vi "LogRelayData.vi"(0 "Path":path, 2 "XCorr":i32, 3 "YCorr":i32, 5 "Rotation":dbl, 7 "Texp":dbl, 9 "CenX":dbl format="%.2f", 11 "CenY":dbl format="%.2g", 13 "XHex":dbl format="%.4f", 14 "YHex":dbl format="%.4f") -> ()   [LabVIEW 2011]
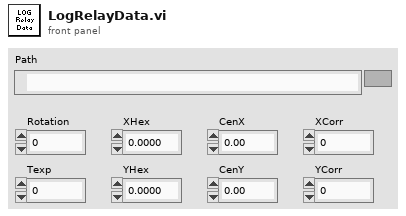
[diagram p1: front panel]
types:
  T1 = enum16{"open", "replace", "create", "open or create", "replace or create", "replace or create with confirmation"}
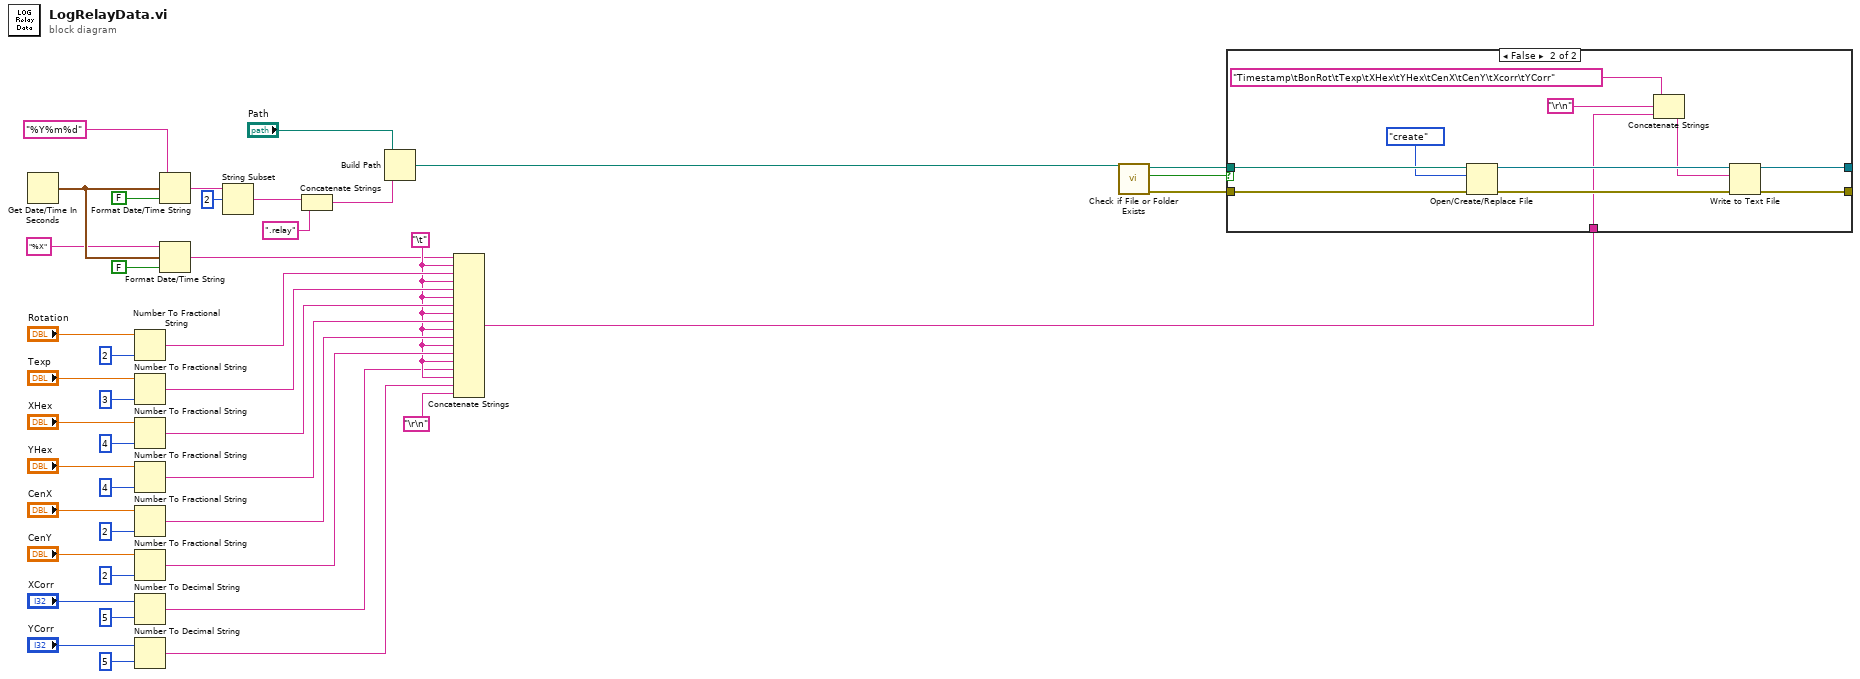
[diagram p0: block diagram]
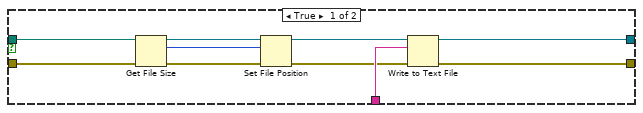
[diagram p2: hidden frame]
diagram:
  w12 = "\t"
  n1 = Get Date/Time In Seconds() -> (seconds since 1Jan1904=w42:timestamp)
  n2 = Number To Fractional String(number="Rotation", precision (6)=i16 2) -> (F-format string=w30:string)  [unwired: 2 in]
  n3 = Number To Fractional String(number="Texp", precision (6)=i16 3) -> (F-format string=w27:string)  [unwired: 2 in]
  n4 = Number To Fractional String(number="XHex", precision (6)=i16 4) -> (F-format string=w16:string)  [unwired: 2 in]
  n5 = Number To Fractional String(number="YHex", precision (6)=i16 4) -> (F-format string=w15:string)  [unwired: 2 in]
  n6 = Number To Fractional String(number="CenX", precision (6)=i16 2) -> (F-format string=w14:string)  [unwired: 2 in]
  n7 = Number To Fractional String(number="CenY", precision (6)=i16 2) -> (F-format string=w13:string)  [unwired: 2 in]
  n8 = Number To Decimal String(number="XCorr", width (-)=i16 5) -> (decimal integer string=w11:string)
  n9 = Number To Decimal String(number="YCorr", width (-)=i16 5) -> (decimal integer string=w10:string)
  n10 = Format Date/Time String(time format string (%c)="%Y%m%d", seconds (now)=w42, UTC format=FALSE) -> (date/time string=w38:string)
  n11 = Format Date/Time String(time format string (%c)="%X", seconds (now)=w42, UTC format=FALSE) -> (date/time string=w2:string)
  n12 = String Subset(string=w38, offset (0)=2) -> (substring=w35:string)  [unwired: 1 in]
  n13 = Concatenate Strings(w35, ".relay" ("string")) -> (w33:string)
  n14 = Build Path(base path="Path", name or relative path=w33) -> (appended path=w5:path)
  n15 = Concatenate Strings(w2, w12, w30, w12, w27, w12, w16, w12, w15, w12, w14, w12, w13, w12, w11, w12, w10, "\r\n") -> (w1:string)
  n16 = call <vilib>:"Check if File or Folder Exists.vi"("path"=w5) -> ("error out"=w8:errorcluster, "file or folder exists?"=w6:bool, "dup path"=w7:path)  [unwired: 8 in]
  n17 = case shown="False" w6 {
    tunnel: w7 -> [w47 w64]
    tunnel: w8 -> [w46 w63]
    tunnel: [w53 w62] -> _
    tunnel: [w52 w61] -> _
    tunnel: w1 -> [w51 w55]
    frame True {
      n18 = Get File Size(file=w47, error in=w46) -> (refnum out=w50:refnum<file>, size (in bytes)=w49:i64, 0:w48:errorcluster)
      n19 = Set File Position(offset (in bytes) (0)=w49, refnum=w50, error in=w48) -> (refnum out=w45:refnum<file>, error out=w44:errorcluster)  [unwired: 1 in]
      n20 = Write to Text File(file (use dialog)=w45, text=w51, error in=w44) -> (refnum out=w53:refnum<file>, error out=w52:errorcluster)  [unwired: 1 in, 1 out]
    }
    frame False {
      n21 = Open/Create/Replace File(file path (use dialog)=w64, error in=w63, operation (0:open)=T1."create") -> (refnum out=w59:refnum<file>, error out=w58:errorcluster)  [unwired: 3 in, 1 out]
      n22 = Concatenate Strings("Timestamp\tBonRot\tTexp\tXHex\tYHex\tCenX\tCenY\tXcorr\tYCorr", "\r\n", w55) -> (w54:string)
      n23 = Write to Text File(file (use dialog)=w59, text=w54, error in=w58) -> (refnum out=w62:refnum<file>, error out=w61:errorcluster)  [unwired: 1 in, 1 out]
    }
  }
